vi "GDSLvClass_StoreClassItemIcon.vi"(0 "Library Refnum":refnum<vi>, 2 "ClassItemIconName":string, 5 "error in (no error)":errorcluster) -> (14 "Library Refnum":refnum<vi>, 19 "error out":errorcluster)   [LabVIEW 2020]
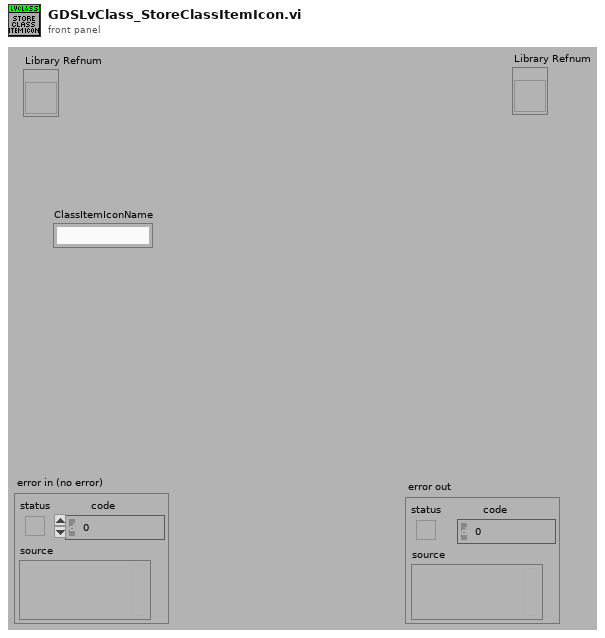
[diagram p1: front panel]
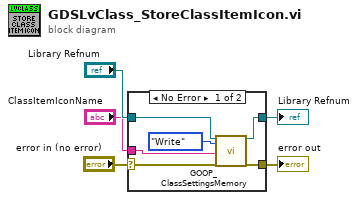
[diagram p0: block diagram]
diagram:
  n1 = case shown="No Error" "error in (no error)" {
    selector: "error in (no error)" -> [w9 w13]
    tunnel: [w6 w13] -> w4
    tunnel: "Library Refnum" -> [w8 w12]
    tunnel: [w7 w12] -> w2
    tunnel: "ClassItemIconName" -> [w10 _]
    frame No Error {
      n2 = call <resource>:"GOOP_ClassSettingsMemory.vi"("Library Refnum"=w8, "Action"=enum16{"Read", "Write"}."Write", "ItemIconIn"=w10, "error in"=w9) -> ("Library Refnum"=w7:refnum<vi>, "error out"=w6:errorcluster)  [unwired: 10 in, 4 out]
    }
    frame Error {
    }
  }
  "Library Refnum" <- w2
  "error out" <- w4
